vi "touchTester.vi"() -> ()   [LabVIEW 2016]
uses:
  <vilib>/NXT/Block Support/NXT_InputPort.ctl
  <vilib>/NXT/Block Support/NXT_OutputPort.ctl
  <vilib>/NXT/NXTIO Xnodes/NXTIONodeSubVIs/NXTMotorRunDistance.vi
  <vilib>/NXT/Dual Mode Library/Waits/Wait_Num.vi
  <vilib>/NXT/Dual Mode Library/Sensors/Touch_Pressed.vi
  <vilib>/NXT/Dual Mode Library/Sensors/EV3_Color_RGB.vi
  <vilib>/NXT/Subs/LVHSConnector.ctl
  <vilib>/NXT/NXTIO Xnodes/AddressXNode/NXTIOAddress.xnode
  <vilib>/NXT/NXTIO Xnodes/NXTIOXNode/NXTIO.xnode
  <vilib>/NXT/LegoClasses/BrickReference/BrickReference.lvclass
panel:
  out "RGB Color":cluster{"Red":u8, "Green":u8, "Blue":u8}
  out "String":string
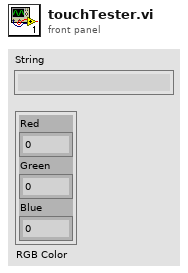
[diagram p1: front panel]
types:
  T1 = typedef "NXT_InputPort.ctl" = u32
  T2 = typedef "NXT_OutputPort.ctl" = u8
  T3 = typedef "LVHSConnector.ctl" = refnum<class "BrickReference.lvclass">
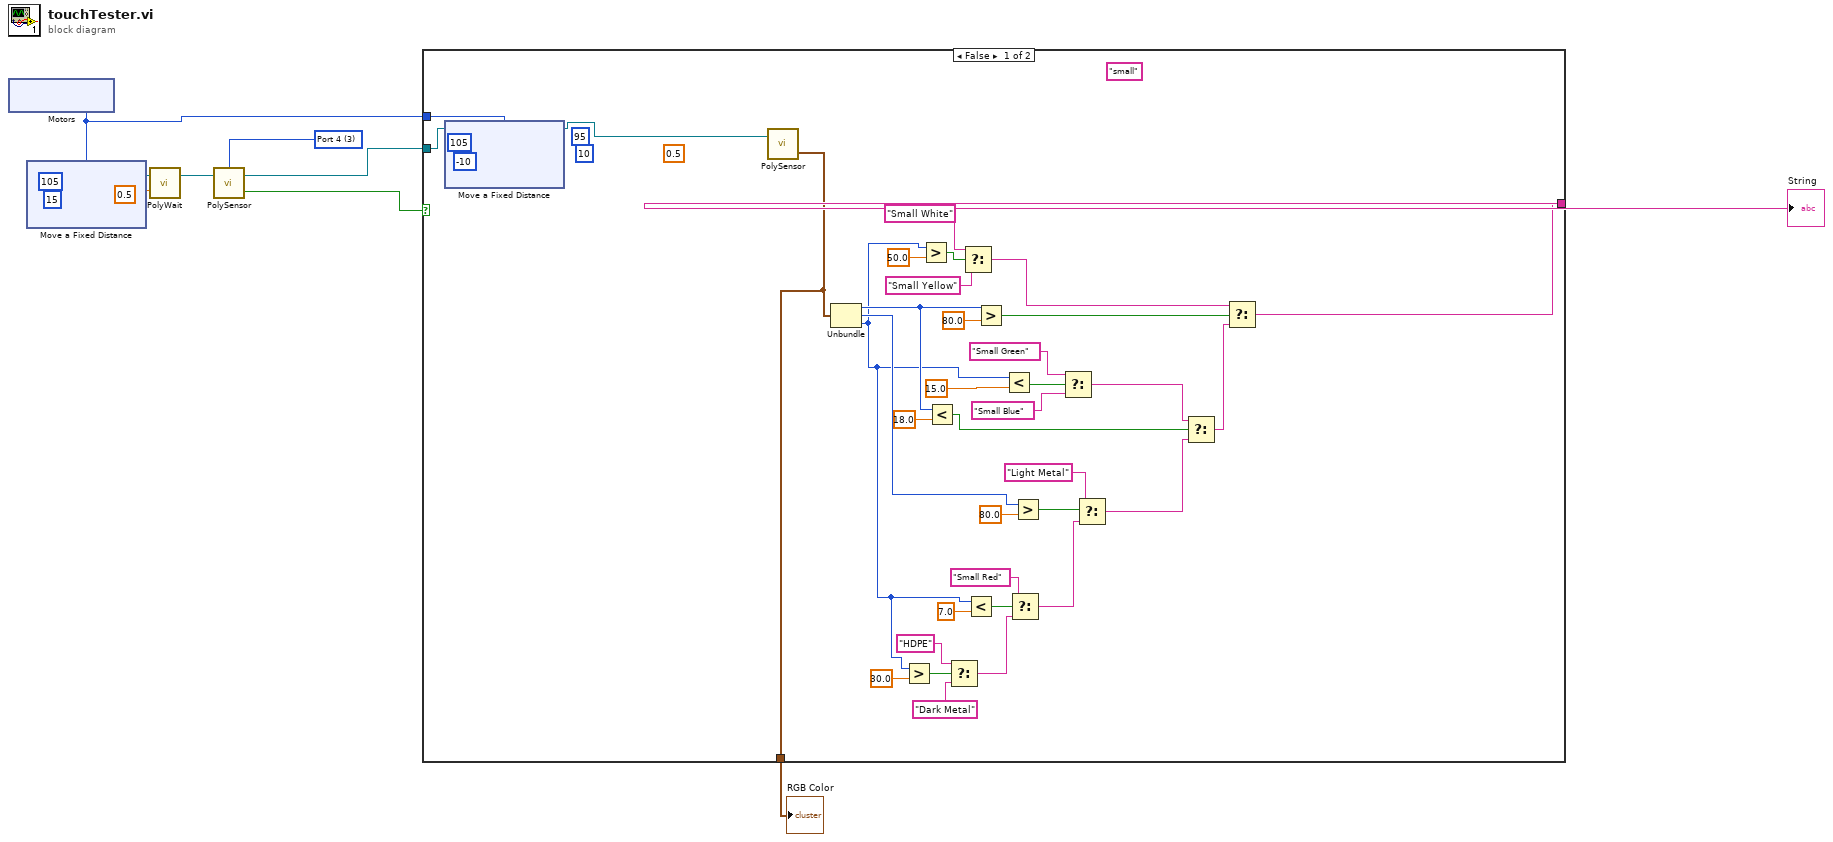
[diagram p0: block diagram]
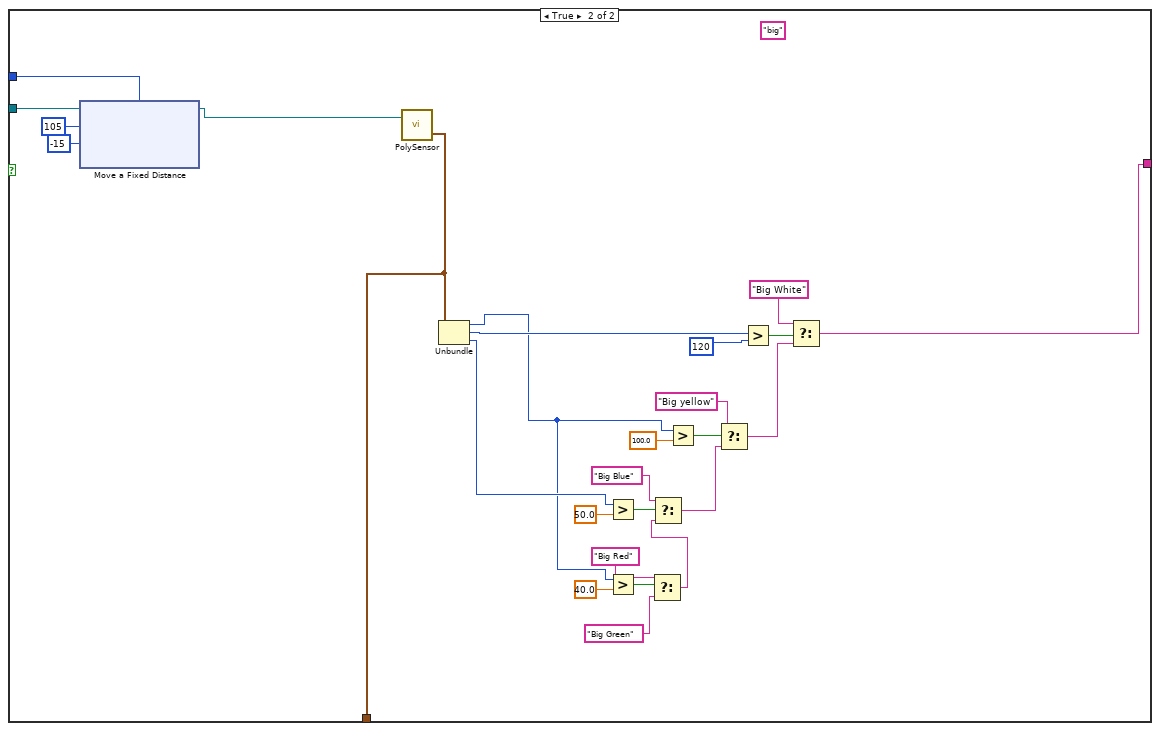
[diagram p2: hidden frame]
diagram:
  w11 = T1 3 items=["Port 1", "Port 2", "Port 3", "Port 4"] ("Port (Port 1)")
  n1 = xnode "Motors"() -> ("Motor"=w3:T2)
  n2 = xnode "Move a Fixed Distance"("Speed 1"=i8 15, "Distance 1"=105, "Motors"=w3) -> ("NXT/EV3"=w9:T3)  [unwired: 2 in]
  n3 = call-poly <vilib>:"PolyWait.vi"("Time (1 sec)"=sgl 0.5, "NXT/EV3"=w9) -> ("NXT/EV3"=w8:T3)  [unwired: 2 in]
  n4 = call-poly <vilib>:"PolySensor.vi"("NXT/EV3"=w8, "Port (Port 1)"=w11) -> ("Yes / No"=w7:bool, "NXT/EV3"=w4:T3)  [unwired: 1 in]
  n5 = case shown="False" w7 {
    tunnel: [w12 w61] -> w6
    tunnel: w4 -> [w47 w84]
    tunnel: w3 -> [w46 w83]
    tunnel: [w44 w81] -> w1
    frame False {
      (unwired) sgl 0.5 ("Time (1 sec)")
      (unwired) 95 ("Distance 1")
      (unwired) i8 10 ("Speed 1")
      (unwired) "small" ("String")
      n6 = xnode "Move a Fixed Distance"("Speed 1"=i8 -10, "Distance 1"=105, "Motors"=w46, "NXT/EV3"=w47) -> ("NXT/EV3"=w45:T3)  [unwired: 1 in]
      n7 = call-poly <vilib>:"PolySensor.vi"("NXT/EV3"=w45) -> ("RGB Color"=w44:cluster{"Red":u8, "Green":u8, "Blue":u8})  [unwired: 2 in, 1 out]
      n8 = Unbundle(w44) -> ("Red"=w35:u8, "Green"=w25:u8, "Blue"=w14:u8)
      n9 = Greater?(x=w14, y=30.0) -> (0:w17:bool)
      n10 = Greater?(x=w14, y=50.0) -> (0:w39:bool)
      n11 = Less?(x=w35, y=18.0) -> (x < y?=w34:bool)
      n12 = Select(t="HDPE", s=w17, f="Dark Metal") -> (s? t:f=w18:string)
      n13 = Select(t="Small White", s=w39, f="Small Yellow") -> (s? t:f=w41:string)
      n14 = Less?(x=w14, y=7.0) -> (x < y?=w21:bool)
      n15 = Greater?(x=w35, y=80.0) -> (0:w43:bool)
      n16 = Less?(x=w14, y=15.0) -> (x < y?=w33:bool)
      n17 = Select(t="Small Red", s=w21, f=w18) -> (s? t:f=w22:string)
      n18 = Greater?(x=w25, y=80.0) -> (0:w26:bool)
      n19 = Select(t="Small Green", s=w33, f="Small Blue") -> (s? t:f=w31:string)
      n20 = Select(t="Light Metal", s=w26, f=w22) -> (s? t:f=w28:string)
      n21 = Select(t=w31, s=w34, f=w28) -> (s? t:f=w23:string)
      n22 = Select(t=w41, s=w43, f=w23) -> (s? t:f=w12:string)
    }
    frame True {
      (unwired) "big"
      n23 = xnode "Move a Fixed Distance"("Speed 1"=i8 -15, "Distance 1"=105, "Motors"=w83, "NXT/EV3"=w84) -> ("NXT/EV3"=w82:T3)  [unwired: 1 in]
      n24 = call-poly <vilib>:"PolySensor.vi"("NXT/EV3"=w82) -> ("RGB Color"=w81:cluster{"Red":u8, "Green":u8, "Blue":u8})  [unwired: 2 in, 1 out]
      n25 = Unbundle(w81) -> ("Red"=w66:u8, "Green"=w78:u8, "Blue"=w71:u8)
      n26 = Greater?(x=w71, y=50.0) -> (0:w70:bool)
      n27 = Greater?(x=w66, y=40.0) -> (0:w65:bool)
      n28 = Select(t="Big Red", s=w65, f="Big Green") -> (s? t:f=w62:string)
      n29 = Select(t="Big Blue", s=w70, f=w62) -> (s? t:f=w68:string)
      n30 = Greater?(x=w66, y=100.0) -> (0:w74:bool)
      n31 = Select(t="Big yellow", s=w74, f=w68) -> (s? t:f=w76:string)
      n32 = Greater?(x=w78, y=120) -> (0:w80:bool)
      n33 = Select(t="Big White", s=w80, f=w76) -> (s? t:f=w61:string)
    }
  }
  "String" <- w6
  "RGB Color" <- w1
